vi "Get Ideal Fundamental and IMD Slopes Core - TOI.vi"(7 "OIP3":dbl, 9 "Target Pin Per Tone (dBm)":dbl, 10 "Target Pout Per Tone (dBm)":dbl, 11 "List of PINs":dbl[](array[numeric])) -> (1 "IMD Slope":dbl[](array[numeric]), 2 "Fundamental Slope":dbl[](array[numeric]), 3 "List of PINs":dbl[](array[numeric]), 5 "IIP3":dbl)   [LabVIEW 2023]
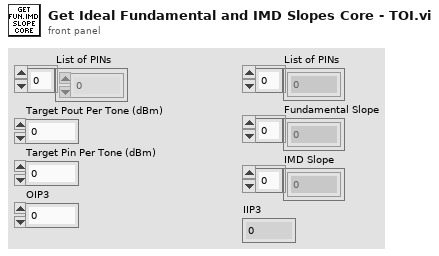
[diagram p1: front panel]
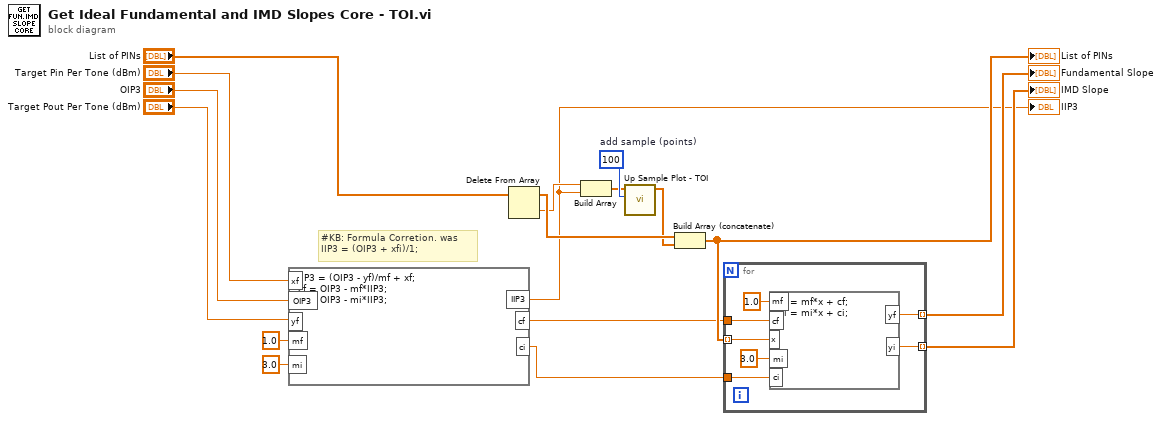
[diagram p0: block diagram]
diagram:
  w9 = 100  # add sample (points)
  # "#KB: Formula Corretion. was \nIIP3 = (OIP3 + xfi)/1;"
  n1 = formula code="IIP3 = (OIP3 - yf)/mf + xf;\ncf = OIP3 - mf*IIP3;\nci = OIP3 - mi*IIP3;"("xf"="Target Pin Per Tone (dBm)", "OIP3"="OIP3", "yf"="Target Pout Per Tone (dBm)", "mf"=1.0 ("input variable"), "mi"=3.0 ("input variable")) -> ("IIP3"=w1:dbl, "cf"=w4:dbl, "ci"=w5:dbl)
  "IIP3" <- w1
  n2 = Delete From Array(array="List of PINs") -> (deleted portion=w12:dbl, array with subset deleted=w14:dbl[])  [unwired: 2 in]
  n3 = Build Array(w12, w1) -> (w8:dbl[])
  n4 = call "Up Sample Plot - TOI.vi"("add N sample between points"=w9, "Plot"=w8) -> ("Ramp Pattern"=w13:dbl[])  [unwired: 9 in]
  n5 = Build Array (concatenate)(w14, w13) -> (w16:dbl[])
  "List of PINs" <- w16
  n6 = for {
    tunnel: w16 -> [w20] mode=indexing
    tunnel: w4 -> [w22]
    tunnel: w5 -> [w21]
    tunnel: [w19] -> w6 mode=indexing
    tunnel: [w18] -> w7 mode=indexing
    n7 = formula code="yf = mf*x + cf;\nyi = mi*x + ci;"("mf"=1.0 ("input variable"), "x"=w20, "mi"=3.0 ("input variable"), "cf"=w22, "ci"=w21) -> ("yf"=w19:dbl, "yi"=w18:dbl)
  }
  "IMD Slope" <- w7
  "Fundamental Slope" <- w6
